vi "Auto cyclic quad ROI.vi"(1 "img_H":i32, 2 "img_W":i32) -> (0 "ROI to crop (pixels)":T1={"Xmax"=2147483647, "Ymax"=2147483647, "Xmin"=0, "Ymin"=0})   [LabVIEW 2018]
uses:
  Typedefs/ROI bounds.ctl
panel:
  in  "Pixel reduction":i32=30
  # "PN 07/12/2015"
  # "Make this value\n30 if using 2mx2m Turntable"
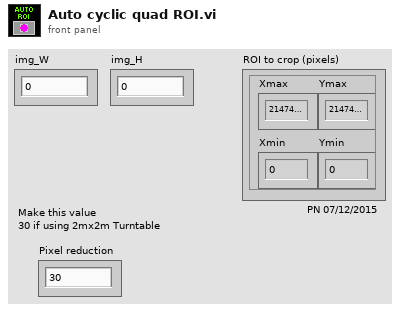
[diagram p1: front panel]
types:
  T1 = typedef "ROI bounds.ctl" = cluster{"Xmax":i32, "Ymax":i32, "Xmin":i32, "Ymin":i32}
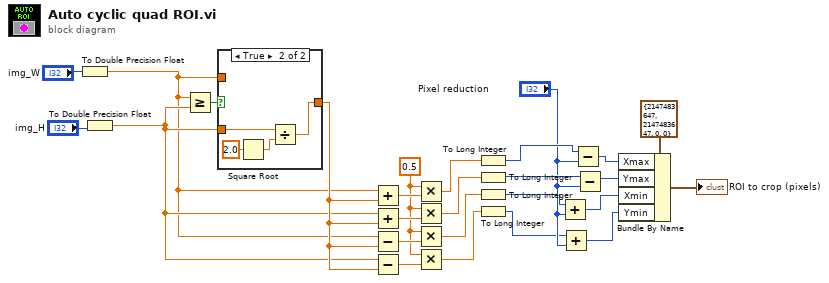
[diagram p0: block diagram]
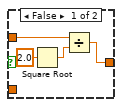
[diagram p2: hidden frame]
diagram:
  w15 = 0.5 ("x")
  n1 = To Double Precision Float(number="img_W") -> (double precision float=w10:dbl)
  n2 = To Double Precision Float(number="img_H") -> (double precision float=w11:dbl)
  n3 = Greater Or Equal?(x=w10, y=w11) -> (x >= y?=w24:bool)
  n4 = case shown="True" w24 {
    tunnel: w10 -> [w28 _]
    tunnel: w11 -> [_ w34]
    tunnel: [w27 w31] -> w18
    frame False {
      n5 = Square Root(x=2.0) -> (sqrt(x)=w30:dbl)
      n6 = Divide(x=w28, y=w30) -> (x/y=w27:dbl)
    }
    frame True {
      n7 = Square Root(x=2.0) -> (sqrt(x)=w33:dbl)
      n8 = Divide(x=w34, y=w33) -> (x/y=w31:dbl)
    }
  }
  n9 = Add(x=w10, y=w18) -> (x+y=w22:dbl)
  n10 = Add(x=w11, y=w18) -> (x+y=w20:dbl)
  n11 = Subtract(x=w10, y=w18) -> (x-y=w17:dbl)
  n12 = Subtract(x=w11, y=w18) -> (x-y=w16:dbl)
  n13 = Multiply(x=w15, y=w22) -> (x*y=w21:dbl)
  n14 = Multiply(x=w15, y=w20) -> (x*y=w19:dbl)
  n15 = Multiply(x=w15, y=w17) -> (x*y=w14:dbl)
  n16 = Multiply(x=w15, y=w16) -> (x*y=w13:dbl)
  n17 = To Long Integer(number=w21) -> (32bit integer=w9:i32)
  n18 = To Long Integer(number=w19) -> (32bit integer=w7:i32)
  n19 = To Long Integer(number=w14) -> (32bit integer=w3:i32)
  n20 = To Long Integer(number=w13) -> (32bit integer=w4:i32)
  n21 = Add(x=w3, y="Pixel reduction") -> (x+y=w2:i32)
  n22 = Add(x=w4, y="Pixel reduction") -> (x+y=w1:i32)
  n23 = Subtract(x=w9, y="Pixel reduction") -> (x-y=w8:i32)
  n24 = Subtract(x=w7, y="Pixel reduction") -> (x-y=w6:i32)
  n25 = Bundle By Name(cluster=T1 {"Xmax"=2147483647, "Ymax"=2147483647, "Xmin"=0, "Ymin"=0} ("ROI to crop (pixels)"), "Xmax"=w8, "Ymax"=w6, "Xmin"=w2, "Ymin"=w1) -> (→"ROI to crop (pixels)":T1)
